vi "DAQ Read.vi"(8 "error in (no error)":errorcluster, 10 "Acquisition and Logging Configuration":T1={"Data Rate (Hz)"=1.0, "Samples per Read"=0, "Number of Reads to Save"=0, "Data File Name"="", "TDMS Properties"=[], "Number of Channels"=4, "Channel Scale Array"=[0.0, 0.0, 0.0, 0.0], "Channel Names"=[], "Trigger - RMS Value"=0.0, "Trigger - Channel"=0, "Trigger - Time (Minute)"=0, "Enable RMS Trigger"=FALSE, "Enable Time Trigger"=FALSE, "Always Log"=FALSE}, 11 "DAQmx Task Name":refnum<k21>) -> (0 "error out":errorcluster, 1 "Waveform Data":waveform(dbl)[](array[waveform]), 2 "dup Acquisition and Logging Configuration":T1={"Data Rate (Hz)"=1.0, "Samples per Read"=0, "Number of Reads to Save"=0, "Data File Name"="", "TDMS Properties"=[], "Number of Channels"=4, "Channel Scale Array"=[0.0, 0.0, 0.0, 0.0], "Channel Names"=[], "Trigger - RMS Value"=0.0, "Trigger - Channel"=0, "Trigger - Time (Minute)"=0, "Enable RMS Trigger"=FALSE, "Enable Time Trigger"=FALSE, "Always Log"=FALSE})   [LabVIEW 2013]
doc: "Reads waveform data from the DAQmx device."
uses:
  Tests/Untitled Project 2/controls/Acquisition and Logging Configuration.ctl
  Tests/Untitled Project 2/controls/TDMS Properties.ctl
  <vilib>/DAQmx/read.llb/DAQmx Read (Analog 1D Wfm NChan NSamp).vi
  Tests/Untitled Project 2/Globals/Global - Monitoring Variables.vi
  <vilib>/DAQmx/miscellaneous.llb/DAQmx Fill In Error Info.vi
  <resource>/objmgr/daqmx.rc
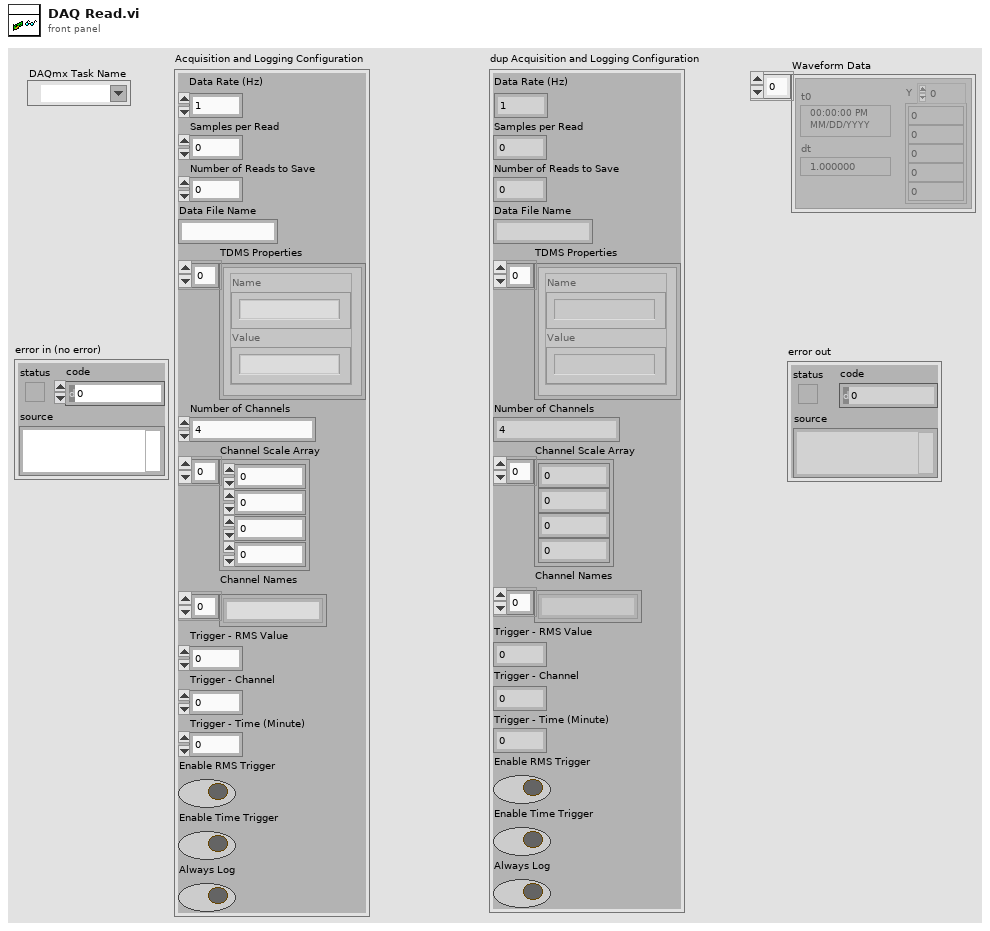
[diagram p1: front panel]
types:
  T1 = typedef "Acquisition and Logging Configuration.ctl" = cluster{"Data Rate (Hz)":dbl, "Samples per Read":i32, "Number of Reads to Save":i32, "Data File Name":string, "TDMS Properties":T2[], "Number of Channels":i32, "Channel Scale Array":dbl[], "Channel Names":string[], "Trigger - RMS Value":dbl, "Trigger - Channel":i32, "Trigger - Time (Minute)":i32, "Enable RMS Trigger":bool, "Enable Time Trigger":bool, "Always Log":bool}
  T2 = typedef "TDMS Properties.ctl" = cluster{"Name":string, "Value":string}
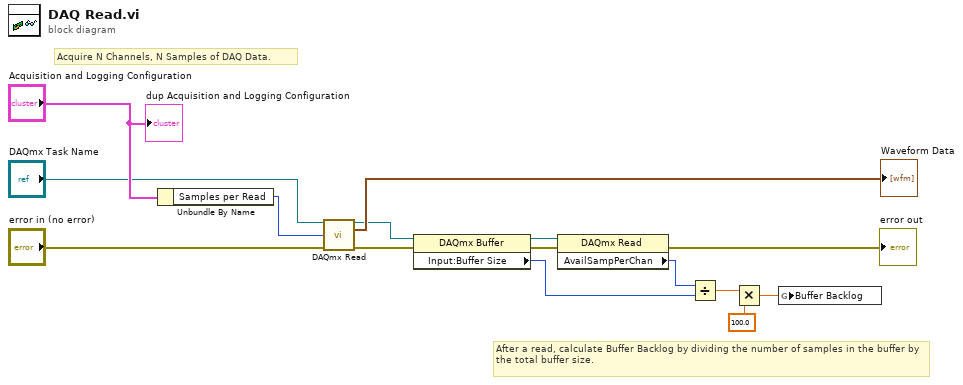
[diagram p0: block diagram]
diagram:
  # "After a read, calculate Buffer Backlog by dividing the number of samples in the buffer by the total buffer size."
  # "Acquire N Channels, N Samples of DAQ Data."
  n1 = Unbundle By Name("Acquisition and Logging Configuration") -> ("Samples per Read"=w13:i32)
  n2 = call-poly <vilib>:"DAQmx Read.vi"("task/channels in"="DAQmx Task Name", "number of samples per channel"=w13, "error in"="error in (no error)") -> ("task out"=w9:refnum<k21>, "data"=→"Waveform Data":waveform(dbl)[], "error out"=w10:errorcluster)  [unwired: 10 in]
  n3 = property class="DAQmx Buffer"(reference=w9, error in=w10) -> (reference out=w7:refnum<k21>, error out=w8:errorcluster, "Input:Buffer Size"=w6:u32)
  n4 = property class="DAQmx Read"(reference=w7, error in=w8) -> (error out=→"error out":errorcluster, "AvailSampPerChan"=w1:u32)  [unwired: 1 out]
  n5 = Divide(x=w1, y=w6) -> (x/y=w4:dbl)
  n6 = Multiply(x=w4, y=100.0) -> (x*y=w3:dbl)
  n7 = global write "Global - Monitoring Variables.vi" "Buffer Backlog"(w3) -> ()
  "dup Acquisition and Logging Configuration" <- "Acquisition and Logging Configuration"
